vi "getObjectList.vi"(4 "error in (no error)":errorcluster) -> (0 "error out":errorcluster, 1 "obj exists":bool, 2 "object names":string[](array[string]), 3 "object refs":refnum<class "HGF_Reference.lvclass">[](array[class]))   [LabVIEW 2012, in "HGF_ObjectManager.lvlib"]
doc: "This VI returns arrays with object references and corresponding names."
uses:
  HGF_ObjectManager.lvlib
  HGF_BaseClasses/HGF_Reference/HGF_Reference.lvclass
  action.ctl
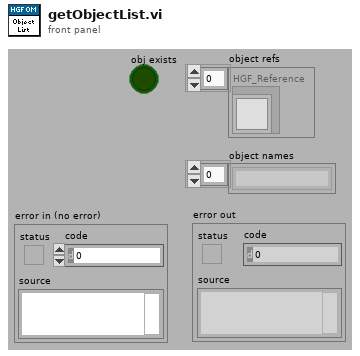
[diagram p1: front panel]
types:
  T1 = typedef "HGF_ObjectManager.lvlib/action.ctl" = enum16{"add", "remove", "name2ref", "ref2name ", "obj exists?", "cleanup", "get object list", "reset"}
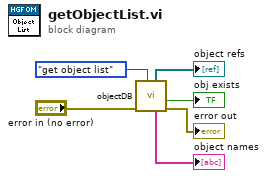
[diagram p0: block diagram]
diagram:
  n1 = call "objectDB.vi"("Action"=action."get object list", "error in (no error)"="error in (no error)") -> ("error out"=→"error out":errorcluster, "obj exists"=→"obj exists":bool, "object list names"=→"object names":string[], "object list refs"=→"object refs":refnum<class "HGF_Reference.lvclass">[])  [unwired: 4 in, 2 out]
